vi "Example - Download with Progress and Abort (RUST).vi"() -> ()   [LabVIEW 2020]
uses:
  <vilib>/Utility/sysdir.llb/System Directory Type.ctl
  Client/Client.lvclass
  Request/Request.lvclass
  ClientBuilder/ClientBuilder.lvclass
  <vilib>/ptbypt/NI_PtbyPt.lvlib
panel:
  out "MB/s":dbl(knob) scale=0.0..20.0
  out "total (ms)":dbl
  out "downloading":bool
  in  "timeout (10000)":i32=10000
  out "complete":bool[](array[boolean])
  in  "Exit":bool
  in  "Start":bool
  in  "Files to Download":string[](array[string])=["http://download.ni.com/evaluation/labview/lvtn/vipm/packages/NI_GDS_2016/NI_GDS_2016-1.1.83.83.vip", "http://download.ni.com/evaluation/labview/lvtn/vipm/packages/ni_gds/ni_gds-1.1.87.94.vip", "http://download.ni.com/evaluation/labview/lvtn/vipm/packages/s5s_aloha/s5s_aloha-2.0.0.22.vip", "http://download.ni.com/evaluation/labview/lvtn/vipm/packages/s5s_aloha_system/s5s_aloha_system-2.0.0.22.vip"]
  out "Progress":dbl[](array[slide]) scale=0.0..100.0
  out "bytes downloaded":u64[](array[numeric])
  out "file size (bytes)":u64[](array[numeric])
  in  "Abort":bool
  in  "Folder to save file(s)":path
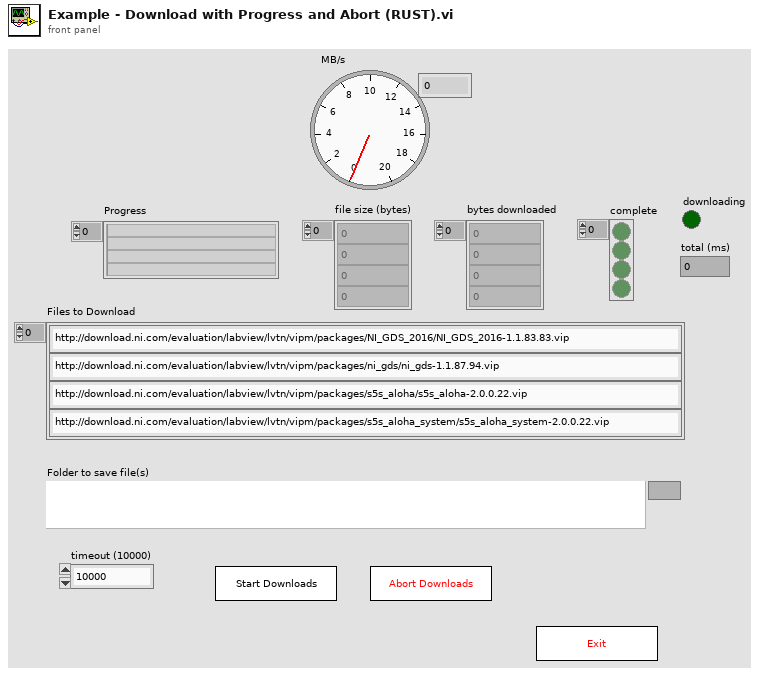
[diagram p1: front panel]
types:
  T1 = typedef "System Directory Type.ctl" = i32
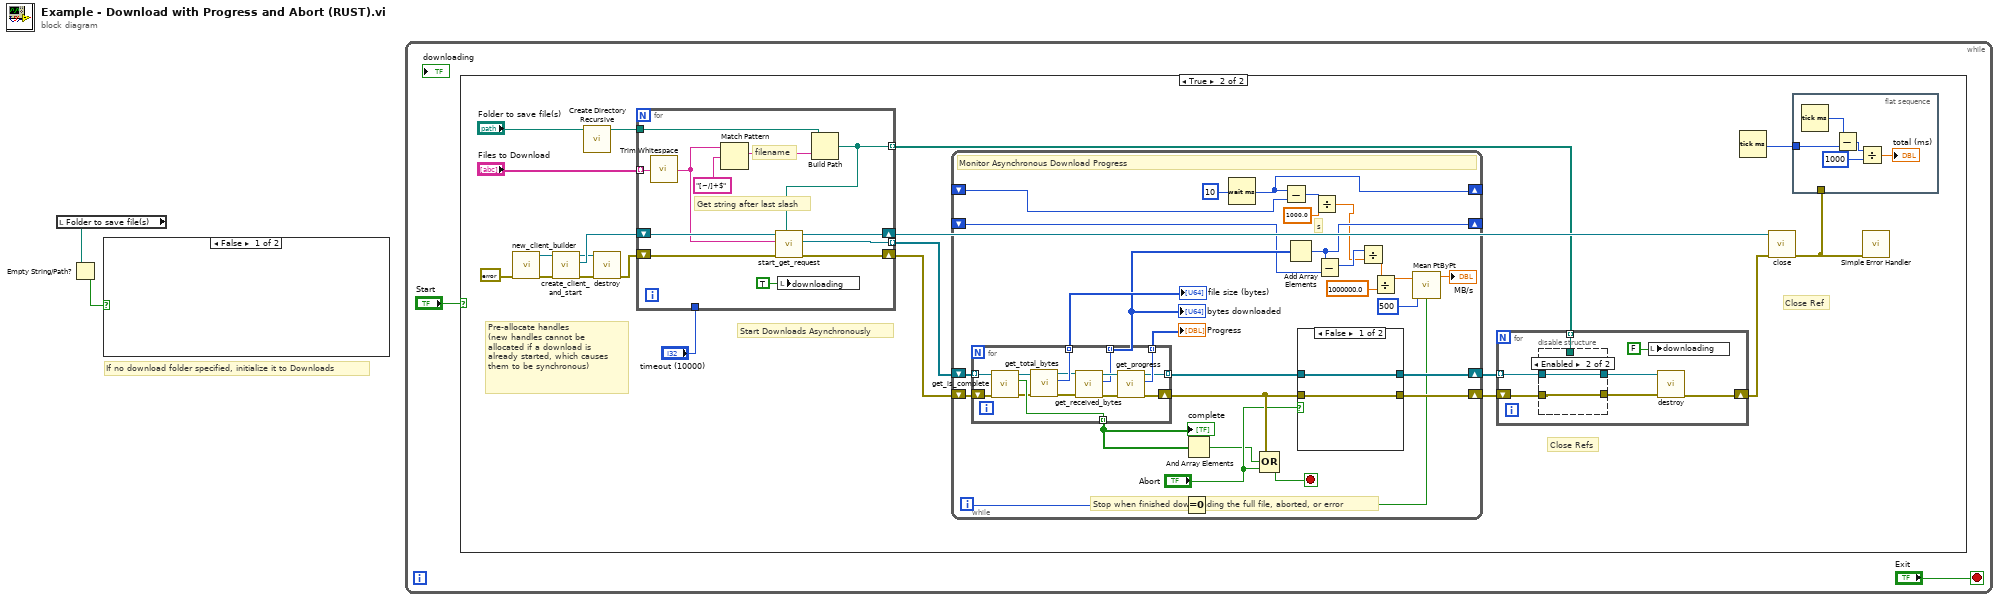
[diagram p0: block diagram]
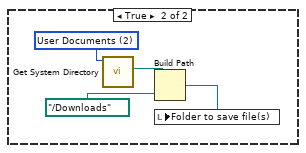
[diagram p2: hidden frame]
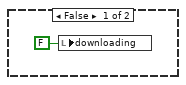
[diagram p3: hidden frame]
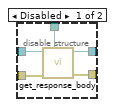
[diagram p4: hidden frame]
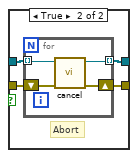
[diagram p5: hidden frame]
diagram:
  # "If no download folder specified, initialize it to Downloads"
  n1 = local read "Folder to save file(s)"() -> (w2:path)
  n2 = Empty String/Path?(string/path=w2) -> (empty?=w1:bool)
  n3 = case shown="False" w1 {
    frame False {
    }
    frame True {
      w6 = T1 2 items=["User Home"=0, "User Desktop"=1, "User Documents"=2, "User Application Data"=3, "User Preferences"=4, "User Temporary"=5, "Public Documents"=6, "Public Application Data"=7, "Public Preferences"=8, "Public Cache"=13, "System Core Libraries"=9, "System Installed Libraries"=10, "Application Files"=11, "Boot Volume Root"=12] ("system directory type")
      n4 = call <vilib>:"Get System Directory.vi"("system directory type"=w6) -> ("system directory"=w5:path)  [unwired: 10 in]
      n5 = Build Path(base path=w5, name or relative path=path "../Downloads" ("base path")) -> (appended path=w3:path)
      n6 = local write "Folder to save file(s)"(w3) -> ()
    }
  }
  n7 = while {
    stop <- "Exit" stop-if-true
    n8 = case shown="True" "Start" {
      frame False {
        n9 = local write "downloading"(FALSE ("downloading")) -> ()
      }
      frame True {
        # "Start Downloads Asynchronously"
        # "Close Ref"
        # "Close Refs"
        # "Pre-allocate handles\n(new handles cannot be allocated if a download is already started, which causes them to be synchronous)"
        n10 = call "new_client_builder.vi"("error in (no error)"=errorcluster {"status"=FALSE, "code"=0, "source"=""} ("error out")) -> ("error out"=w17:errorcluster, "Client out"=w18:refnum<class "ClientBuilder.lvclass">)  [unwired: 9 in]
        n11 = call "create_client_and_start.vi"("error in"=w17, "ClientBuilder in"=w18) -> ("error out"=w11:errorcluster, "Client out"=w16:refnum<class "Client.lvclass">, "ClientBuilder out"=w12:refnum<class "ClientBuilder.lvclass">)  [unwired: 7 in]
        n12 = call <vilib>:"Create Directory Recursive.vi"("directory"="Folder to save file(s)") -> ("directory copy"=w13:path)  [unwired: 4 in, 2 out]
        n13 = call "destroy.vi"("error in (no error)"=w11, "ClientBuilder in"=w12) -> ("error out"=w10:errorcluster)  [unwired: 9 in]
        n14 = for {
          tunnel: w13 -> [w58]
          tunnel: [w52] -> w26 mode=indexing
          tunnel: "Files to Download" -> [w57] mode=indexing
          shift-right: [w51] -> w29
          shift-left: w10 -> [w54]
          tunnel: "timeout (10000)" -> [_]
          shift-right: [w50] -> w23
          shift-left: w16 -> [w55]
          tunnel: [w49] -> w19 mode=indexing
          # "Get string after last slash"
          # "filename"
          n15 = call <vilib>:"Trim Whitespace.vi"("string"=w57) -> ("trimmed string"=w53:string)  [unwired: 1 in]
          n16 = Match Pattern(string=w53, regular expression="[~/]+$") -> (match substring=w59:string)  [unwired: 1 in, 3 out]
          n17 = local write "downloading"(TRUE ("downloading")) -> ()
          n18 = Build Path(base path=w58, name or relative path=w59) -> (appended path=w49:path)
          n19 = call "start_get_request.vi"("save_to_file"=w49, "error in (no error)"=w54, "url"=w53, "Client in"=w55) -> ("error out"=w51:errorcluster, "Request"=w52:refnum<class "Request.lvclass">, "Client out"=w50:refnum<class "Client.lvclass">)  [unwired: 5 in]
        }
        n20 = while {
          shift-right: [w86] -> w27
          shift-left: w29 -> [w87]
          shift-right: [w82] -> w28
          shift-left: w26 -> [w88]
          shift-right: [w75] -> _
          shift-left: _ -> [w74]
          shift-right: [w67] -> _
          shift-left: _ -> [w72]
          i -> [w63]
          stop <- w89 stop-if-true
          # "s"
          # "Stop when finished downloading the full file, aborted, or error"
          # "Monitor Asynchronous Download Progress"
          n21 = for {
            tunnel: w88 -> [w102] mode=indexing
            tunnel: [w95] -> w76 mode=indexing
            tunnel: [w94] -> w81 mode=indexing
            tunnel: [w99] -> w83 mode=indexing
            tunnel: [w100] -> w78 mode=indexing
            tunnel: [w101] -> w80 mode=indexing
            shift-right: [w98] -> w85
            shift-left: w87 -> [w103]
            n22 = call "get_is_complete.vi"("error in (no error)"=w103, "Request in"=w102) -> ("error out"=w90:errorcluster, "is_complete"=w101:bool, "Request out"=w93:refnum<class "Request.lvclass">)  [unwired: 7 in]
            n23 = call "get_total_bytes.vi"("error in (no error)"=w90, "Request in"=w93) -> ("error out"=w91:errorcluster, "total_bytes"=w94:u64, "Request out"=w92:refnum<class "Request.lvclass">)  [unwired: 7 in]
            n24 = call "get_received_bytes.vi"("error in (no error)"=w91, "Request in"=w92) -> ("error out"=w96:errorcluster, "received_bytes"=w95:u64, "Request out"=w97:refnum<class "Request.lvclass">)  [unwired: 7 in]
            n25 = call "get_progress.vi"("error in (no error)"=w96, "Request in"=w97) -> ("error out"=w98:errorcluster, "progress"=w100:i32, "Request out"=w99:refnum<class "Request.lvclass">)  [unwired: 7 in]
          }
          "bytes downloaded" <- w76
          "file size (bytes)" <- w81
          "Progress" <- w78
          "complete" <- w80
          n26 = Equal To 0?(x=w63) -> (x = 0?=w62:bool)
          n27 = And Array Elements(Boolean array=w80) -> (logical AND=w79:bool)
          n28 = Wait (ms)(milliseconds to wait=u32 10) -> (millisecond timer value=w67:u32)
          n29 = Compound Arithmetic op=OR(w85, w79, "Abort") -> (w89:bool)
          n30 = Subtract(x=w67, y=w72) -> (x-y=w68:u32)
          n31 = Add Array Elements(numeric array=w76) -> (sum=w75:u64)
          n32 = case shown="False" "Abort" {
            tunnel: [w105 w109] -> w86
            tunnel: w85 -> [w105 w108]
            tunnel: w83 -> [w104 w107]
            tunnel: [w104 w106] -> w82
            frame False {
            }
            frame True {
              # "Abort"
              n33 = for {
                shift-right: [w110] -> w109
                shift-left: w108 -> [w113]
                tunnel: w107 -> [w112] mode=indexing
                tunnel: [w111] -> w106 mode=indexing
                n34 = call "cancel.vi"("error in (no error)"=w113, "Request in"=w112) -> ("error out"=w110:errorcluster, "Request out"=w111:refnum<class "Request.lvclass">)  [unwired: 7 in, 1 out]
              }
            }
          }
          n35 = Divide(x=w68, y=1000.0) -> (x/y=w66:dbl)
          n36 = Subtract(x=w75, y=w74) -> (x-y=w73:u64)
          n37 = Divide(x=w73, y=w66) -> (x/y=w70:dbl)
          n38 = Divide(x=w70, y=1000000.0) -> (x/y=w65:dbl)
          n39 = call <vilib>:"Mean PtByPt.vi"("x"=w65, "sample length"=500, "initialize"=w62) -> ("mean"=→"MB/s":dbl)  [unwired: 1 in, 1 out]
        }
        n40 = for {
          tunnel: w28 -> [w38] mode=indexing
          shift-right: [w40] -> w22
          shift-left: w27 -> [w39]
          tunnel: w19 -> [w35] mode=indexing
          n41 = disable-structure shown="Enabled" {
            disable-tunnel: w39 -> [w46 w47]
            disable-tunnel: w38 -> [w45 w48]
            disable-tunnel: [w44 w48] -> w37
            disable-tunnel: [w43 w47] -> w36
            disable-tunnel: w35 -> [w42 _]
            frame Disabled {
              n42 = call "get_response_body.vi"("save_to_file"=w42, "error in (no error)"=w46, "Request in"=w45) -> ("error out"=w43:errorcluster, "Request in"=w44:refnum<class "Request.lvclass">)  [unwired: 6 in, 1 out]
            }
            frame Enabled {
            }
          }
          n43 = local write "downloading"(FALSE ("downloading")) -> ()
          n44 = call "destroy.vi"("error in (no error)"=w36, "Request in"=w37) -> ("error out"=w40:errorcluster)  [unwired: 8 in, 1 out]
        }
        n45 = Tick Count (ms)() -> (millisecond timer value=w20:u32)
        n46 = call "close.vi"("error in (no error)"=w22, "Client in"=w23) -> ("error out"=w21:errorcluster)  [unwired: 9 in]
        n47 = flat-sequence {
          tunnel: w21 -> [_]
          tunnel: w20 -> [w33]
          frame #0 {
            n48 = Tick Count (ms)() -> (millisecond timer value=w34:u32)
            n49 = Subtract(x=w34, y=w33) -> (x-y=w32:u32)
            n50 = Divide(x=w32, y=u32 1000) -> (x/y=→"total (ms)":dbl)
          }
        }
        n51 = call <vilib>:"Simple Error Handler.vi"("error in (no error)"=w21) -> ()  [unwired: 4 in, 5 out]
      }
    }
  }
